vi "AFM Control.vi"() -> ()   [LabVIEW 2020, in "AFM Control.lvclass"]
doc: "Use this VI to help configure your experiment.\n1. Choose Pickering or Not Pickering\n2. Configure the Electrode control to show which electrode is connected to which lockin\n3. Choose a Label for each electrode to configure Krohn Hite amplifier automatically\n4. Easily set all Krohn Hite channels to be \"all ground\" or \"all differential\" mode\n5. Fill out information about you and your device in the lower left corner\n6. When you are finished, or when you want to update the amplifiers, click the \"CREATE OUTPUT\" button located in upper right. Clicking this button will set the amplifiers, Pickering switch (if you have one), and write information to a functional global variable that you can easily read from elsewhere in your program"
uses:
  AFM Control.lvclass
  Typedefs/Instrument--enum.ctl
  AFM Control.lvclass/AFM Control.ctl
  <userlib>/_MGI/File/MGI Create Directory Chain Behavior Enum.ctl
  <vilib>/MakerHub/Toolbox/LMH-Toolbox.lvlib
panel:
  in  "Create Output":bool
  in  "OK":bool
  out "Control Experiment":refnum<class "AFM Control.lvclass">
  in  "Control Experiment":refnum<class "AFM Control.lvclass">
  in  "Tab Control":T1(tab)=enum."LevyLabVIEW output"
  in  "Project & Device Description":string="this is a test"
  in  "Sample":string="TEST"
  in  "Device":string="20191017"
  in  "Instrument":T2=enum."EBL"
  in  "Username":string="Dengyu"
  out "device":string="TEST.20191017"
  out "comments":string="Device: \r  Device Name: TEST.20191017\r  Computer: BLACKPEARL\r  User: Dengyu\r  Instrument: EBL\r  Description: |\r    this is a test\r\rExperiment: \r  Time: 2019-10-18T11:10:03\r  Description: |\rSweep: \r- Loop1: [OFF, 0.000000]\r- Loop2: [OFF, 0.000000]\r- Loop3: [OFF, 0.000000]\r- Loop4: [OFF, 0.000000]\r\rWiring: \r- Electrode 1: Lockin 1, I-, KH1 Channel 1, Differential, 1x, 50k Ohms\r- Electrode 2: Lockin 2, Vsg, KH1 Channel 2, Differential, 1x, 50k Ohms\r- Electrode 4: Lockin 3, V1+, KH1 Channel 3, SE+ (-gnd), 10x, Open\r- Electrode 3: Lockin 4, V1-, KH1 Channel 4, SE+ (-gnd), 10x, Open\r- Electrode 26: Lockin 6, I+, KH1 Channel 6, Differential, 1x, 50k Ohms\r\rLockin: \r  AO: \r  - AO 1: amp = 10.000 mV, DC = 0.000 mV, f = 13.00 Hz, phi = 0.00°, Sine\r  - AO 2: amp = 0.000 mV, DC = 0.000 mV, f = 13.00 Hz, phi = 0.00°, Sine\r  - AO 3: amp = 0.000 mV, DC = 0.000 mV, f = 13.00 Hz, phi = 0.00°, Sine\r  - AO 4: amp = 0.000 mV, DC = 0.000 mV, f = 13.00 Hz, phi = 0.00°, Sine\r  REF: \r  - Lockin 1: f = 13.00 Hz, phi = 0.00°, TC = 0.10 s, order = 2 \r  Sampling: \r  - Fs: 65000.000000\r  - N: 5000\r"
  out "folder":string="G:\\My Drive\\ansom\\Data\\EBL\\TEST.20191017" caption="(\\base path\\project\\device\\ )"
  out "Values have changed":bool
  in  "KH Same Gain":bool
  in  "KH Same Shunt":bool
  out "YAML example":string="description: This is a dummy dataset which mimics smFRET data.\n\nsetup:\n    ## Mandatory fields\n    num_pixels: 2                # using 2 detectors\n    num_spots: 1                 # a single confocal excitation\n    num_spectral_ch: 2           # donor and acceptor detection\n    num_polarization_ch: 1       # no polarization selection\n    num_split_ch: 1              # no beam splitter\n    modulated_excitation: False  # CW excitation, no modulation\n    lifetime: False              # no TCSPC in detection\n\n    ## Optional fields\n    excitation_wavelengths:      # List of excitation wavelenghts\n       - !!float 532e-9\n    excitation_cw:               # List of booleans, True if wavelength is CW\n       - True\n    detection_wavelengths:       # Nominal center wavelength for each for detection ch\n       - !!float 580e-9\n       - !!float 640e-9\n\nsample:\n  sample_name: describe the sample here\n  buffer_name: describe the buffer here\n  dye_names: 'Cy3B, ATTO647N'   # Comma separates names of fluorophores\n\nidentity:\n    author: Author Name\n    author_affiliation: Name of Research Institution\n\nprovenance:\n    filename: 'photon_data.hdf5'\n    software: Acquisition Software Name\n\nphoton_data:\n    timestamps_specs:\n        timestamps_unit: !!float 10e-9  # 10 ns\n    measurement_specs:\n        measurement_type: smFRET\n        detectors_specs:\n            spectral_ch1: [0]  # list of donor's detector IDs\n            spectral_ch2: [1]  # list of acceptor's detector IDs"
  in  "String":string
  # "Lockin"
  # "Krohn Hite"
  # "Other"
  # "Wiring"
  # "Use this VI to help configure your experiment.\n1. Choose Pickering or Not Pickering\n2. Configure the Electrode control to show which electrode is connected to which lockin\n3. Choose a Label for each electrode to configure Krohn Hite amplifier automatically\n4. Easily set all Krohn Hite channels to be \"all ground\" or \"all differential\" mode\n5. Fill out information about you and your device in the lower left corner\n6. When you are finished, or when you want to update the amplifiers, click the \"CREATE OUTPUT\" button located in upper right.\nClicking this button will set the amplifiers, Pickering switch (if you have one), and write information to a functional global variable that you can easily read from elsewhere in your program"
  # "If you want to have new labels for the \"Labels\" field you can type them here"
  # "Not used:"
  # "The magic words are:\nI\nVsg\nVbg\ndV\nV"
  # "Sample"
  # "Krohn Hite"
  # "Lockin"
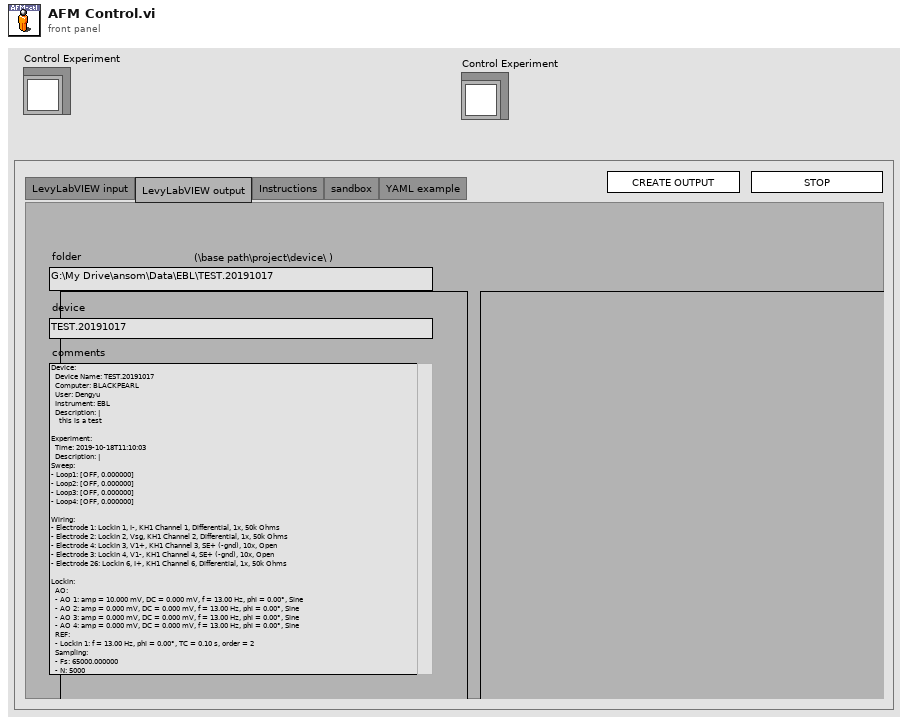
[diagram p1: front panel]
types:
  T1 = enum32{"LevyLabVIEW input", "LevyLabVIEW output", "Instructions", "sandbox", "YAML example"}
  T2 = typedef "AFM Control.lvclass/Instrument--enum.ctl" = enum16{"PPMS", "PPMS2", "MFP3D", "CYPHER", "THz1", "THz2", "MNK", "CF900", "JEOL", "AGILENT", "EBL"}
  T3 = enum32{"invalid app kind", "Development System", "Run Time System", "Student Edition", "Embedded LabVIEW", "Evaluation", "Custom"}
  T4 = enum32{"Invalid", "Standard", "Closed", "Hidden", "Minimized", "Maximized"}
  T5 = typedef "MGI Create Directory Chain Behavior Enum.ctl" = enum16{"Auto Detect", "Path Contains a File", "Path Does Not Contain a File"}
  T6 = typedef "AFM Control.lvclass/Experiment Description--cluster.ctl" = cluster{"User":string, "Device":string, "Device Path":path, "Device Description":string, "Experiment Path":path, "Experiment Description":string, "Instrument":T2}
  T7 = cluster{"Core":cluster{"Current VI Reference":refnum<vi>, "Close Panel on Exit?":bool}, "Control Experiment":refnum<class "AFM Control.lvclass">, "Experiment":T6}
  T8 = cluster{"Current VI Reference":refnum<vi>, "Close Panel on Exit?":bool}
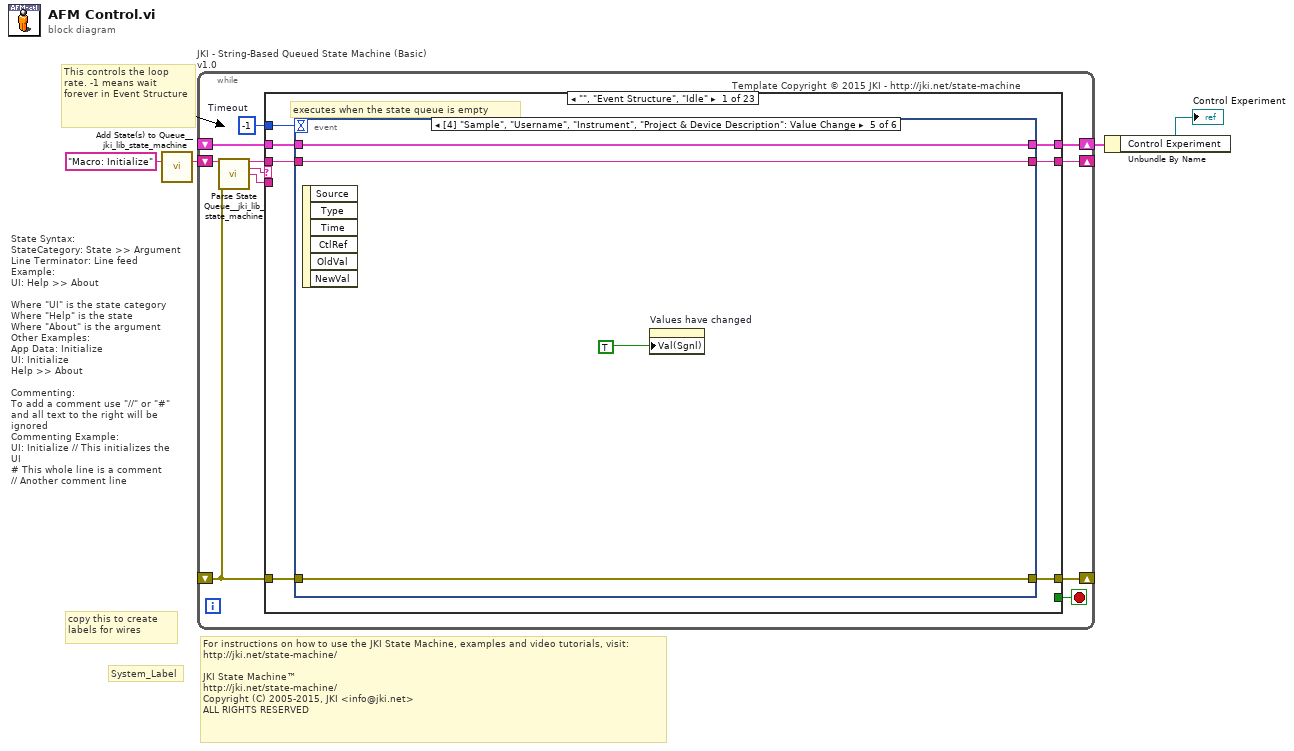
[diagram p0: block diagram]
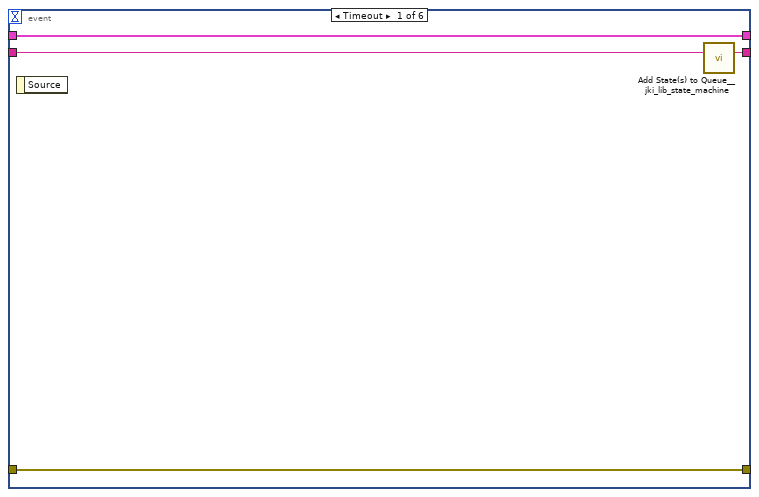
[diagram p2: hidden frame]
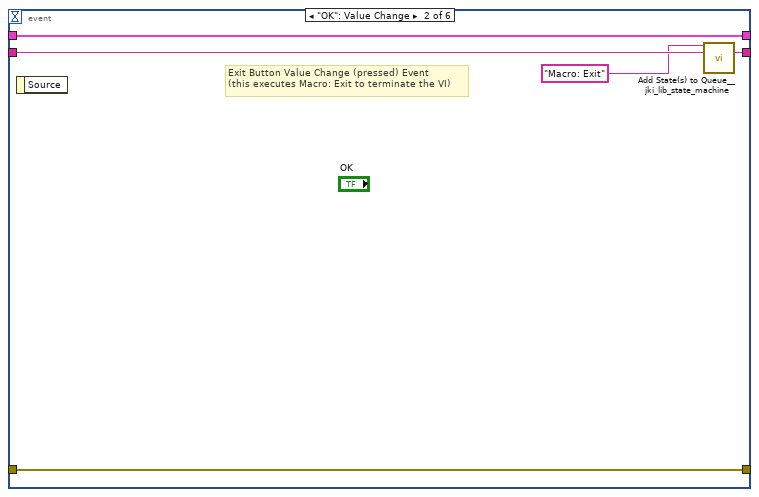
[diagram p3: hidden frame]
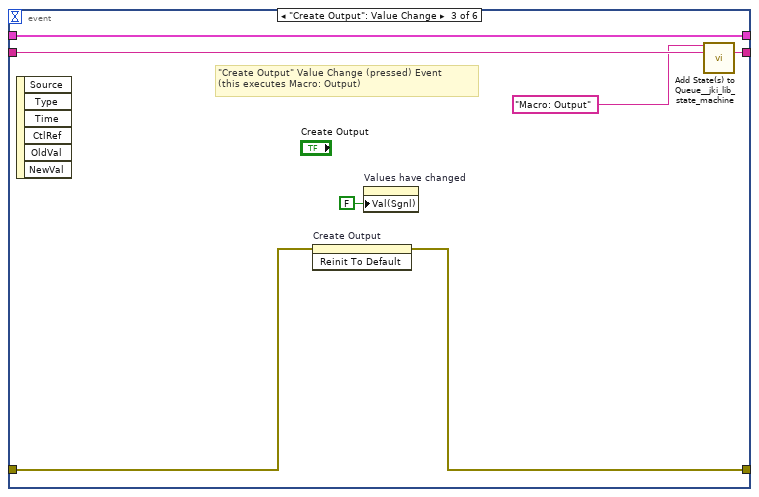
[diagram p4: hidden frame]
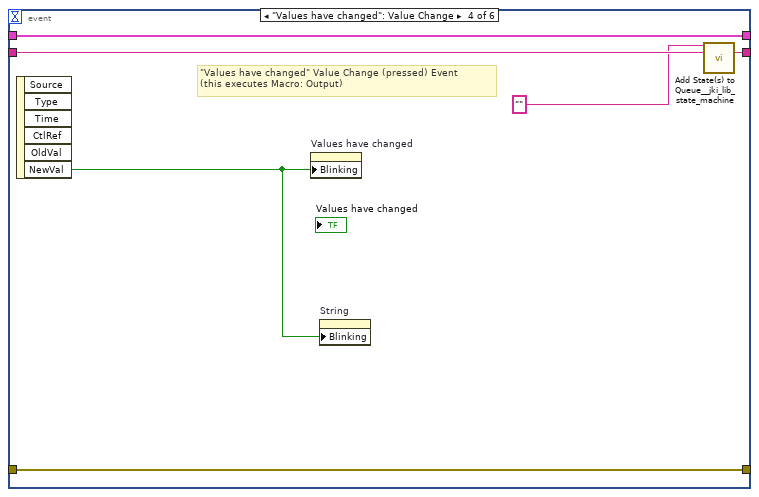
[diagram p5: hidden frame]
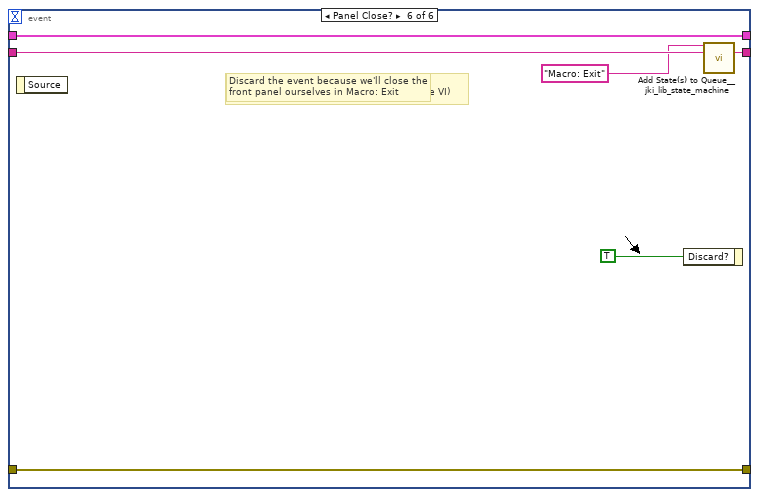
[diagram p6: hidden frame]
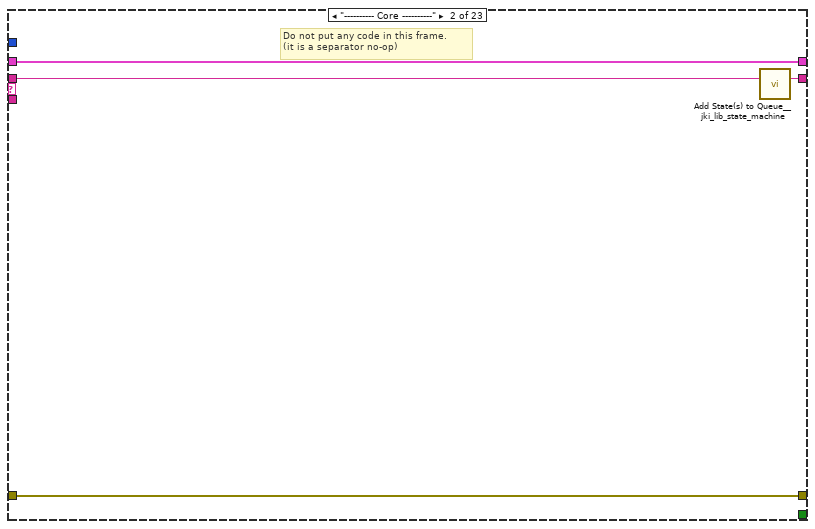
[diagram p7: hidden frame]
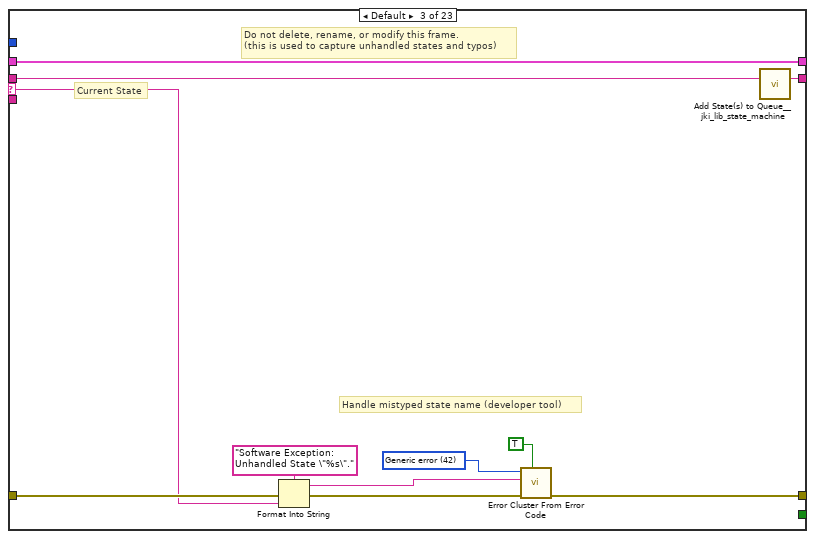
[diagram p8: hidden frame]
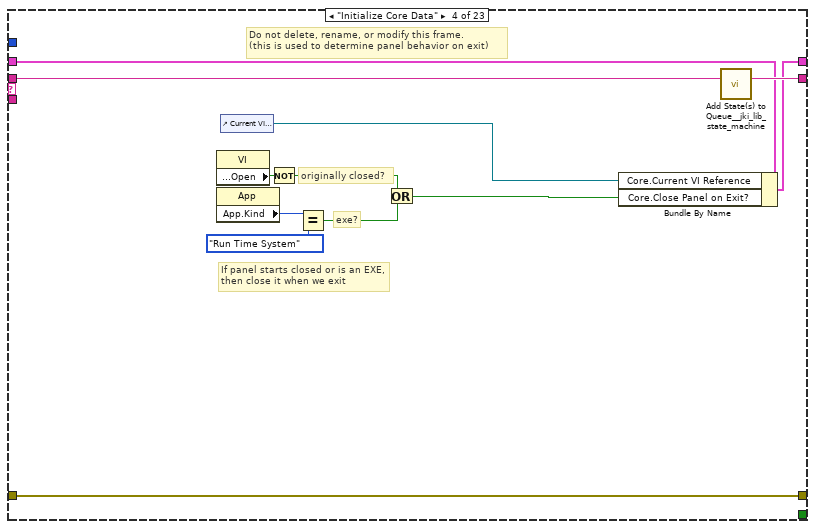
[diagram p9: hidden frame]
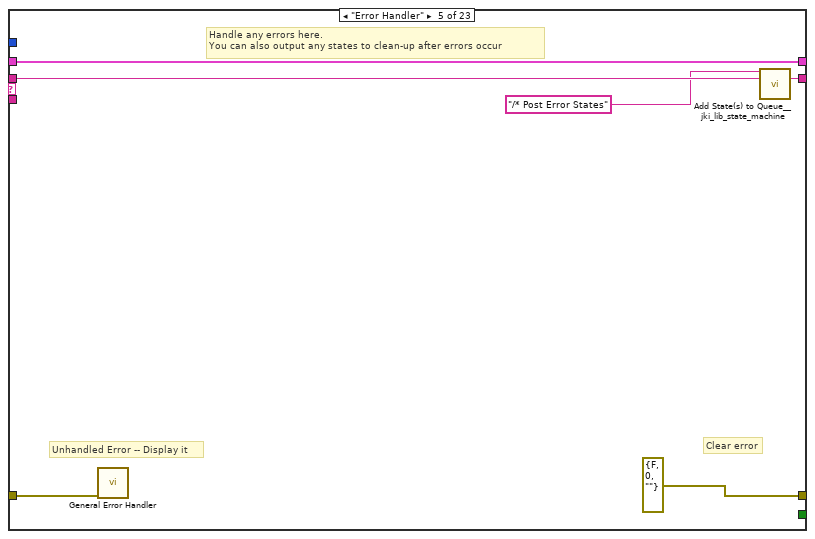
[diagram p10: hidden frame]
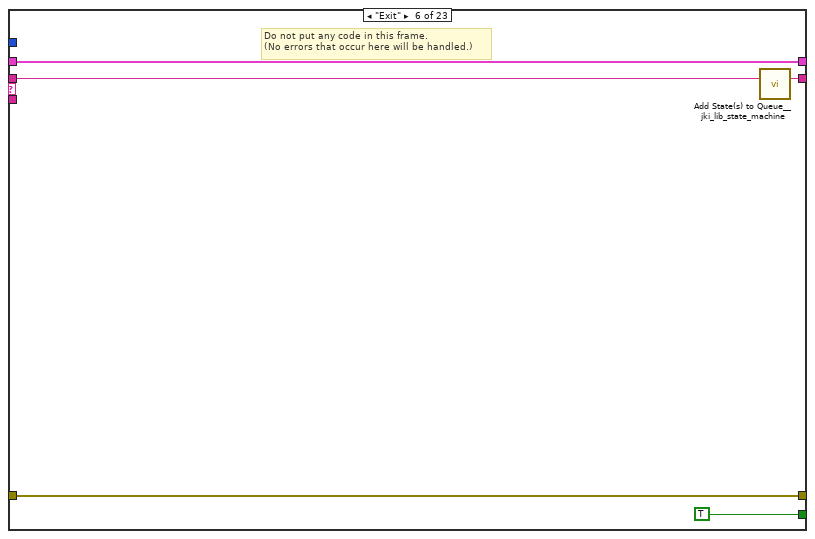
[diagram p11: hidden frame]
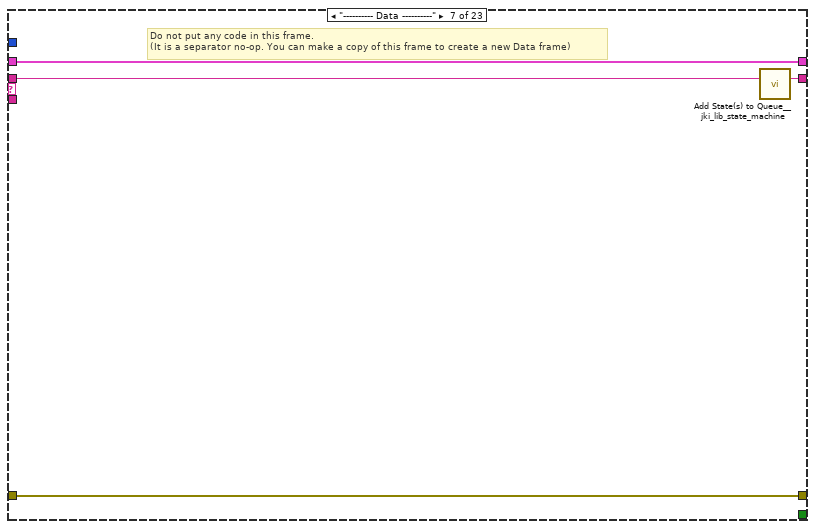
[diagram p12: hidden frame]
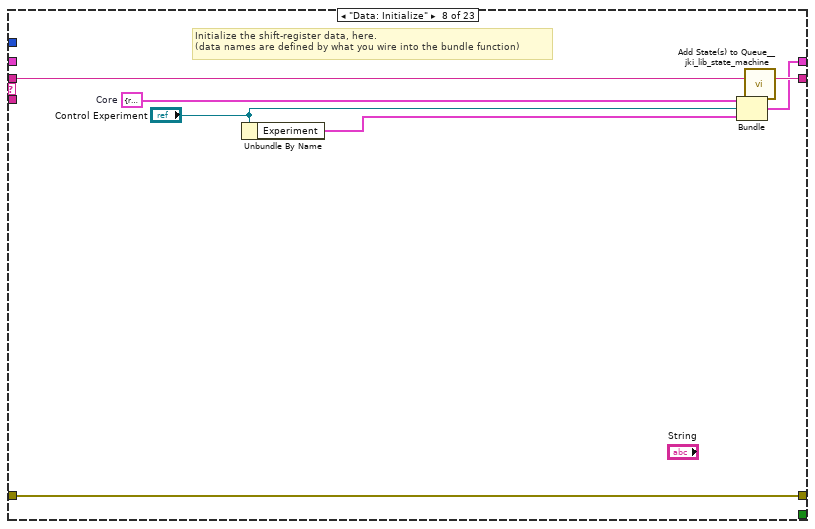
[diagram p13: hidden frame]
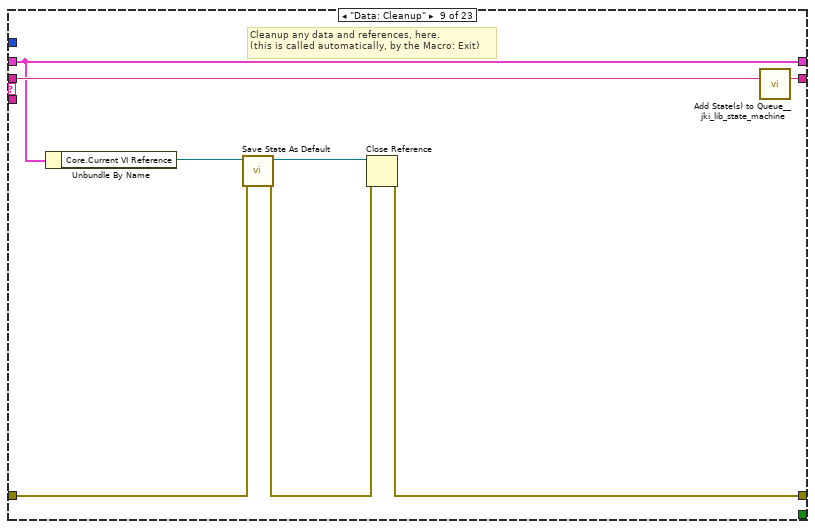
[diagram p14: hidden frame]
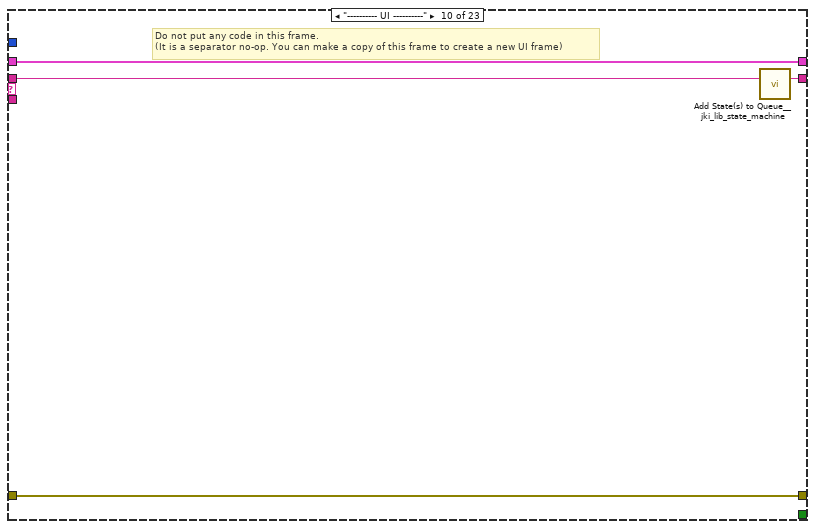
[diagram p15: hidden frame]
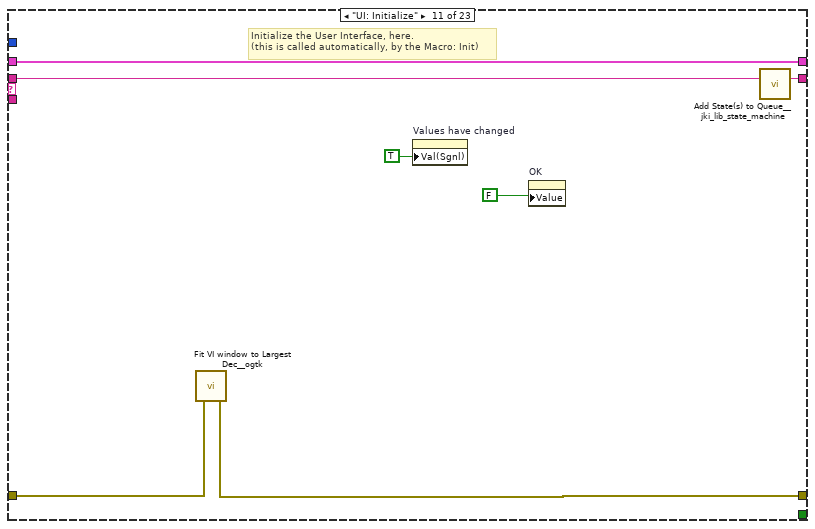
[diagram p16: hidden frame]
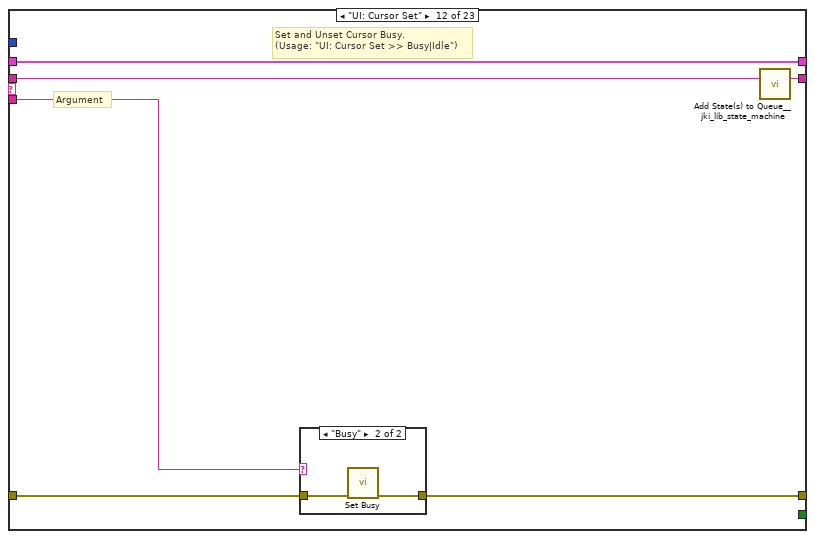
[diagram p17: hidden frame]
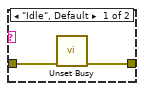
[diagram p18: hidden frame]
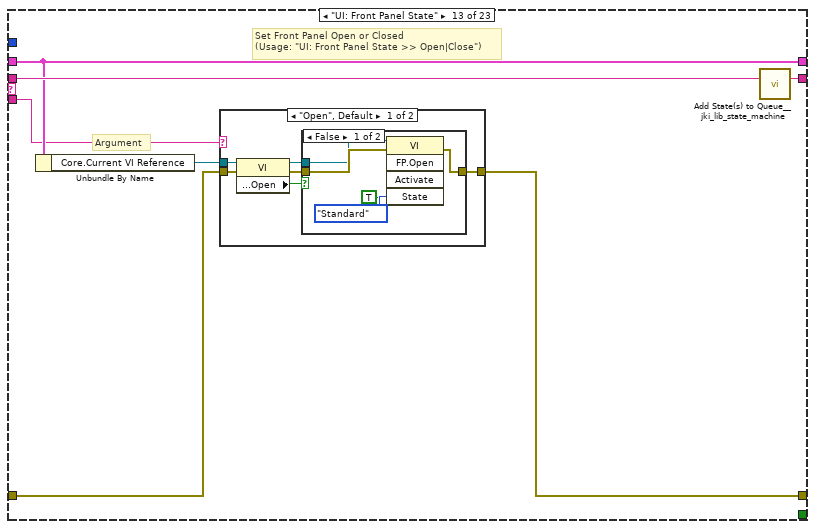
[diagram p19: hidden frame]
diagram:
  # "For instructions on how to use the JKI State Machine, examples and video tutorials, visit:\nhttp://jki.net/state-machine/\n\nJKI State Machine™\nhttp://jki.net/state-machine/\nCopyright (C) 2005-2015, JKI <info@jki.net>\nALL RIGHTS RESERVED"
  # "State Syntax:\nStateCategory: State >> Argument\nLine Terminator: Line feed\nExample:\nUI: Help >> About\n\nWhere \"UI\" is the state category\nWhere \"Help\" is the state\nWhere \"About\" is the argument\nOther Examples:\nApp Data: Initialize\nUI: Initialize\nHelp >> About\n\nCommenting:\nTo add a comment use \"//\" or \"#\" and all text to the right will be ignored\nCommenting Example:\nUI: Initialize // This initializes the UI\n# This whole line is a comment\n// Another comment line"
  # "copy this to create labels for wires"
  # "This controls the loop rate. -1 means wait forever in Event Structure"
  # "System_Label"
  n1 = call <vilib>:"Add State(s) to Queue__jki_lib_state_machine.vi"("State(s) in (\"\")"="Macro: Initialize") -> ("States Out"=w4:string)  [unwired: 14 in]
  n2 = while "JKI - String-Based Queued State Machine (Basic) v1.0" {
    shift-right: [w8] -> w2
    shift-left: _ -> [w7]
    shift-right: [w11] -> _
    shift-left: _ -> [w5]
    shift-right: [w10] -> _
    shift-left: w4 -> [w12]
    stop <- w9 stop-if-true
    w6 = -1  # Timeout
    # "Template Copyright © 2015 JKI - http://jki.net/state-machine"
    n3 = call <vilib>:"Parse State Queue__jki_lib_state_machine.vi"("State Queue"=w12, "Error In (no error)"=w5) -> ("Remaining States"=w14:string, "Current State"=w15:string, "Arguments"=w13:string)  [unwired: 11 in]
    n4 = case shown="\"\", \"Event Structure\", \"Idle\"" w15 {
      selector: w15 -> [_ _ w59 _ _ _ _ _ _ _ _ _ _ _ _ _ _ _ _ _ _ _ _]
      tunnel: w14 -> [w22 w58 w63 w81 w87 w92 w96 w103 w111 w115 w122 w128 w139 w165 w169 w174 w185 w192 w196 w208 w223 w236 w243]
      tunnel: w13 -> [_ _ _ _ _ _ _ _ _ _ _ w123 w133 _ _ _ _ _ _ _ _ _ _]
      tunnel: w7 -> [w20 w55 w61 w72 w84 w90 w93 _ w109 w112 w120 w126 w135 w162 w166 w171 w182 w190 w193 w204 w221 w234 w241]
      tunnel: [w19 w56 w65 w78 errorcluster {"status"=FALSE, "code"=0, "source"=""} ("error out") w89 w94 w100 w108 w113 w116 w124 w136 w163 w167 w172 w183 w187 w194 w206 w211 w227 w239] -> w11
      tunnel: w5 -> [w18 w56 w64 w78 w83 w89 w94 w100 w105 w113 w119 w125 w137 w163 w167 w172 w183 w187 w194 w206 w212 w228 w237]
      tunnel: [w21 w57 w62 w80 w86 w91 w95 w102 w110 w114 w121 w127 w138 w164 w168 w173 w184 w191 w195 w207 w222 w235 w242] -> w10
      tunnel: [_ _ _ _ _ TRUE _ _ _ _ _ _ _ _ _ _ _ _ _ _ _ _ _] -> w9
      tunnel: [w17 w55 w61 w79 w84 w90 w93 w101 w109 w112 w120 w126 w135 w162 w166 w171 w182 w190 w193 w205 w220 w233 w241] -> w8
      tunnel: w6 -> [w16 _ _ _ _ _ _ _ _ _ _ _ _ _ _ _ _ _ _ _ _ _ _]
      frame "", "Event Structure", "Idle" {
        # "executes when the state queue is empty"
        n5 = event shown="[4] \"Sample\", \"Username\", \"Instrument\", \"Project & Device Description\": Value Change" {
          selector: _ -> [_ _ _ _ _ _]
          dyn-events: _ -> [_ _ _ _ _ _]
          timeout: w16 -> [_ _ _ _ _ _]
          tunnel: w22 -> [w26 w31 w38 w44 w46 w54]
          tunnel: [w25 w30 w37 w43 w46 w53] -> w21
          tunnel: w20 -> [w23 w28 w36 w42 w47 w51]
          tunnel: [w24 w29 w33 w40 w48 w52] -> w19
          tunnel: w18 -> [w24 w29 w34 w40 w48 w52]
          tunnel: [w23 w28 w36 w42 w47 w51] -> w17
          event Timeout {
            n6 = event-data() -> ()  [unwired: 1 in, 1 out]
            n7 = call <vilib>:"Add State(s) to Queue__jki_lib_state_machine.vi"("State(s) in (\"\")"=w26) -> ("States Out"=w25:string)  [unwired: 14 in]
          }
          event "OK": Value Change {
            # "Exit Button Value Change (pressed) Event\n(this executes Macro: Exit to terminate the VI)"
            n8 = event-data() -> ()  [unwired: 1 in, 1 out]
            n9 = call <vilib>:"Add State(s) to Queue__jki_lib_state_machine.vi"("State(s) in Front (\"\")"="Macro: Exit", "State(s) in (\"\")"=w31) -> ("States Out"=w30:string)  [unwired: 13 in]
          }
          event "Create Output": Value Change {
            # "\"Create Output\" Value Change (pressed) Event\n(this executes Macro: Output)"
            n10 = event-data() -> ()  [unwired: 1 in, 6 out]
            n11 = invoke on="Create Output" class="Bool" method="Reinit To Default"(error in=w34) -> (error out=w33:errorcluster)  [unwired: 2 in, 2 out]
            n12 = property on="Values have changed" class="Bool (strict)"("Val(Sgnl)"=FALSE ("Value (Signaling)")) -> ()  [unwired: 2 in, 2 out]
            n13 = call <vilib>:"Add State(s) to Queue__jki_lib_state_machine.vi"("State(s) in Front (\"\")"="Macro: Output", "State(s) in (\"\")"=w38) -> ("States Out"=w37:string)  [unwired: 13 in]
          }
          event "Values have changed": Value Change {
            # "\"Values have changed\" Value Change (pressed) Event\n(this executes Macro: Output)"
            n14 = event-data() -> ("NewVal"=w39:bool)  [unwired: 1 in, 5 out]
            n15 = property on="Values have changed" class="Bool (strict)"("Blinking"=w39) -> ()  [unwired: 2 in, 2 out]
            n16 = property on="String" class="Str"("Blinking"=w39) -> ()  [unwired: 2 in, 2 out]
            n17 = call <vilib>:"Add State(s) to Queue__jki_lib_state_machine.vi"("State(s) in Front (\"\")"="", "State(s) in (\"\")"=w44) -> ("States Out"=w43:string)  [unwired: 13 in]
          }
          event "Sample", "Username", "Project & Device Description": Value Change {
            n18 = event-data() -> ()  [unwired: 1 in, 6 out]
            n19 = property on="Values have changed" class="Bool (strict)"("Val(Sgnl)"=TRUE ("Values have changed")) -> ()  [unwired: 2 in, 2 out]
          }
          event Panel Close? {
            # "Discard the event because we'll close the front panel ourselves in Macro: Exit"
            # "Close Panel button (pressed) Event\n(this executes Macro: Exit to terminate the VI)"
            n20 = event-data() -> ()  [unwired: 1 in, 1 out]
            n21 = event-data("Discard?"=TRUE) -> ()  [unwired: 1 in, 1 out]
            n22 = call <vilib>:"Add State(s) to Queue__jki_lib_state_machine.vi"("State(s) in Front (\"\")"="Macro: Exit", "State(s) in (\"\")"=w54) -> ("States Out"=w53:string)  [unwired: 13 in]
          }
        }
      }
      frame "---------- Core ----------" {
        # "Do not put any code in this frame.\n(it is a separator no-op)"
        n23 = call <vilib>:"Add State(s) to Queue__jki_lib_state_machine.vi"("State(s) in (\"\")"=w58) -> ("States Out"=w57:string)  [unwired: 14 in]
      }
      frame Default {
        w68 = 42 items=["No error", "Argument error", "Memory is full", "Out of zone", "End of file", "File already open", "Generic file I/O error", "File not found", "File permission error", "Disk is full", "Duplicate path", "Too many files open", "System feature not enabled", "Resource file not found", "Cannot add resource", "Resource not found", "Image not found", "Image memory error", "Pen does not exist", "Config type invalid", "Config token not found", "Config parse error", "Config memory error", "Bad external code format", "Bad external code offset", "External code not present", "Null window", "Destroy window error", "Null menu", "Print aborted", "Bad print record", "Print driver error", "Windows error during printing", "Memory error during printing", "Print dialog error", "Generic print error", "Invalid device refnum", "Device not found", "Device parameter error", "Device unit error", "Cannot open device", "Device call aborted", "Generic error", "Cancelled by user", "Object ID too low", "Object ID too high", "Object not in heap", "Unknown heap", "Unknown object (invalid DefProc)", "Unknown object (DefProc not in table)", "Message out of range", "Invalid (null) method", "Unknown message", "Manager call not supported", "Bad address", "Network operation in progress", "Network operation timed out", "Connection is busy", "Network attribute not supported", "Network error", "Address in use", "System out of memory", "Connection aborted", "Connection refused", "Not connected", "Already connected", "Connection closed", "Initialization error (interapplication manager)", "Bad occurrence", "Wait on unbound occurrence handler", "Occurrence queue overflow", "Datalog type conflict", "Unused", "Unrecognized type (interapplication manager)", "Memory corrupt", "Failed to make temporary DLL", "Old CIN version", "Drag socket not found", "Failed to load drop-object", "Failed to register OLE object", "Failed to release OLE object", "Format specifier type mismatch", "Unknown format specifier", "Too few format specifiers", "Too many format specifiers", "Scan failed", "Newer CIN version", "Error converting to variant", "Runtime menu error", "Password tampered", "Variant attribute not found", "Incompatible variant data type", "Event data is not available", "Event Store is not present", "Occurrence is not found", "Event Queue is not created", "Event info is not available", "Refnum passed is NULL", "Error retrieving Class GUID", "Error retrieving CoClass GUID", "Error retrieving TypeLib GUID.", "Bad built application magic bytes.", "Specific driver is different from the specific driver associated with the Logical Name.", "There is no session opened to the class driver.", "Max Error", "MAX - Error with config objects", "MAX - Error loading configuration", "MAX - Group not supported"]
        # "Current State"
        # "Do not delete, rename, or modify this frame.\n(this is used to capture unhandled states and typos)"
        # "Handle mistyped state name (developer tool)"
        n24 = Format Into String(format string="Software Exception: Unhandled State \"%s\"." ("message"), error in=w64, w59) -> (resulting string=w67:string, error out=w66:errorcluster)  [unwired: 1 in]
        n25 = call <vilib>:"Error Cluster From Error Code.vi"("show call chain? (False)"=TRUE, "error in (no error)"=w66, "error message (\"\")"=w67, "error code (0)"=w68) -> ("error out"=w65:errorcluster)  [unwired: 5 in]
        n26 = call <vilib>:"Add State(s) to Queue__jki_lib_state_machine.vi"("State(s) in (\"\")"=w63) -> ("States Out"=w62:string)  [unwired: 14 in]
      }
      frame "Initialize Core Data" {
        # "Do not delete, rename, or modify this frame.\n(this is used to determine panel behavior on exit)"
        # "originally closed?"
        # "exe?"
        # "If panel starts closed or is an EXE, then close it when we exit"
        n27 = property class="VI"() -> ("Front Panel.Open"=w77:bool)  [unwired: 2 in, 2 out]
        n28 = property class="App"() -> ("App.Kind"=w76:T3)  [unwired: 2 in, 2 out]
        n29 = control-ref of="Current VI Reference"() -> (w70:refnum<vi>)
        n30 = Not(x=w77) -> (.not. x?=w74:bool)
        n31 = Equal?(x=w76, y=T3."Run Time System" ("Application:Kind")) -> (x = y?=w73:bool)
        n32 = Or(x=w74, y=w73) -> (x .or. y?=w71:bool)
        n33 = Bundle By Name(cluster=w72, "Core.Current VI Reference"=w70, "Core.Close Panel on Exit?"=w71) -> (w79:T7)
        n34 = call <vilib>:"Add State(s) to Queue__jki_lib_state_machine.vi"("State(s) in (\"\")"=w81) -> ("States Out"=w80:string)  [unwired: 14 in]
      }
      frame "Error Handler" {
        # "Unhandled Error -- Display it"
        # "Handle any errors here.\nYou can also output any states to clean-up after errors occur"
        # "Clear error"
        n35 = call <vilib>:"General Error Handler.vi"("error in (no error)"=w83) -> ()  [unwired: 10 in, 5 out]
        n36 = call <vilib>:"Add State(s) to Queue__jki_lib_state_machine.vi"("State(s) in Front (\"\")"="/* Post Error States", "State(s) in (\"\")"=w87) -> ("States Out"=w86:string)  [unwired: 13 in]
      }
      frame "Exit" {
        # "Do not put any code in this frame.\n(No errors that occur here will be handled.)"
        n37 = call <vilib>:"Add State(s) to Queue__jki_lib_state_machine.vi"("State(s) in (\"\")"=w92) -> ("States Out"=w91:string)  [unwired: 14 in]
      }
      frame "---------- Data ----------" {
        # "Do not put any code in this frame.\n(It is a separator no-op. You can make a copy of this frame to create a new Data frame)"
        n38 = call <vilib>:"Add State(s) to Queue__jki_lib_state_machine.vi"("State(s) in (\"\")"=w96) -> ("States Out"=w95:string)  [unwired: 14 in]
      }
      frame "Data: Initialize" {
        w99 = T8 {"Current VI Reference"=refnum, "Close Panel on Exit?"=FALSE}  # Core
        # "Initialize the shift-register data, here.\n(data names are defined by what you wire into the bundle function)"
        n39 = Unbundle By Name("Control Experiment") -> ("Experiment"=w97:T6)
        n40 = Bundle("Core"=w99, "Control Experiment"="Control Experiment", "Experiment"=w97) -> (w101:T7)  [unwired: 1 in]
        n41 = call <vilib>:"Add State(s) to Queue__jki_lib_state_machine.vi"("State(s) in (\"\")"=w103) -> ("States Out"=w102:string)  [unwired: 14 in]
      }
      frame "Data: Cleanup" {
        # "Cleanup any data and references, here.\n(this is called automatically, by the Macro: Exit)"
        n42 = Unbundle By Name(w109) -> ("Core.Current VI Reference"=w107:refnum<vi>)
        n43 = call <vilib>:"Save State As Default.vi"("Error In"=w105, "Target VI"=w107) -> ("Error Out"=w104:errorcluster, "Target VI"=w106:refnum<vi>)  [unwired: 8 in]
        n44 = Close Reference(reference=w106, error in (no error)=w104) -> (error out=w108:errorcluster)
        n45 = call <vilib>:"Add State(s) to Queue__jki_lib_state_machine.vi"("State(s) in (\"\")"=w111) -> ("States Out"=w110:string)  [unwired: 14 in]
      }
      frame "---------- UI ----------" {
        # "Do not put any code in this frame.\n(It is a separator no-op. You can make a copy of this frame to create a new UI frame)"
        n46 = call <vilib>:"Add State(s) to Queue__jki_lib_state_machine.vi"("State(s) in (\"\")"=w115) -> ("States Out"=w114:string)  [unwired: 14 in]
      }
      frame "UI: Initialize" {
        # "Initialize the User Interface, here.\n(this is called automatically, by the Macro: Init)"
        n47 = call <userlib>:"Fit VI window to Largest Dec__ogtk.vi"("error in (no error)"=w119) -> ("error out"=w116:errorcluster)  [unwired: 5 in, 1 out]
        n48 = property on="Values have changed" class="Bool (strict)"("Val(Sgnl)"=TRUE ("Blinking")) -> ()  [unwired: 2 in, 2 out]
        n49 = property on="OK" class="Bool (strict)"("Value"=FALSE ("Blinking")) -> ()  [unwired: 2 in, 2 out]
        n50 = call <vilib>:"Add State(s) to Queue__jki_lib_state_machine.vi"("State(s) in (\"\")"=w122) -> ("States Out"=w121:string)  [unwired: 14 in]
      }
      frame "UI: Cursor Set" {
        # "Argument"
        # "Set and Unset Cursor Busy.\n(Usage: \"UI: Cursor Set >> Busy|Idle\")"
        n51 = case shown="\"Busy\"" w123 {
          tunnel: w125 -> [w130 w132]
          tunnel: [w129 w131] -> w124
          frame "Idle", Default {
            n52 = call <vilib>:"Unset Busy.vi"("error in (no error)"=w130) -> ("error out"=w129:errorcluster)  [unwired: 10 in]
          }
          frame "Busy" {
            n53 = call <vilib>:"Set Busy.vi"("error in (no error)"=w132) -> ("error out"=w131:errorcluster)  [unwired: 9 in, 1 out]
          }
        }
        n54 = call <vilib>:"Add State(s) to Queue__jki_lib_state_machine.vi"("State(s) in (\"\")"=w128) -> ("States Out"=w127:string)  [unwired: 14 in]
      }
      frame "UI: Front Panel State" {
        # "Argument"
        # "Set Front Panel Open or Closed\n(Usage: \"UI: Front Panel State >> Open|Close\")"
        n55 = Unbundle By Name(w135) -> ("Core.Current VI Reference"=w134:refnum<vi>)
        n56 = case shown="\"Open\", Default" w133 {
          tunnel: w137 -> [w143 w156]
          tunnel: [w145 w157] -> w136
          tunnel: w134 -> [w144 w154]
          frame "Open", Default {
            n57 = property class="VI"(reference=w144, error in=w143) -> (reference out=w141:refnum<vi>, error out=w142:errorcluster, "Front Panel.Open"=w140:bool)
            n58 = case shown="False" w140 {
              tunnel: [w148 w151] -> w145
              tunnel: w142 -> [w147 w151]
              tunnel: w141 -> [w146 _]
              frame False {
                n59 = invoke class="VI" method="FP.Open"(reference=w146, error in=w147, "Activate"=TRUE, "State"=T4."Standard") -> (error out=w148:errorcluster)  [unwired: 1 in, 4 out]
              }
              frame True {
              }
            }
          }
          frame "Close" {
            n60 = property class="VI"(reference=w154, error in=w156) -> (reference out=w153:refnum<vi>, error out=w155:errorcluster, "Front Panel.Open"=w152:bool)
            n61 = case shown="True" w152 {
              tunnel: [w158 w161] -> w157
              tunnel: w155 -> [w158 w160]
              tunnel: w153 -> [_ w159]
              frame False {
              }
              frame True {
                n62 = invoke class="VI" method="FP.Close"(reference=w159, error in=w160) -> (error out=w161:errorcluster)  [unwired: 1 in, 2 out]
              }
            }
          }
        }
        n63 = call <vilib>:"Add State(s) to Queue__jki_lib_state_machine.vi"("State(s) in (\"\")"=w139) -> ("States Out"=w138:string)  [unwired: 14 in]
      }
      frame "UI: Buttons" {
        # "Do not put any code in this frame.\n(It is a separator no-op. You can make a copy of this frame to create a new UI frame)"
        n64 = call <vilib>:"Add State(s) to Queue__jki_lib_state_machine.vi"("State(s) in (\"\")"=w165) -> ("States Out"=w164:string)  [unwired: 14 in]
      }
      frame "---------- Macro ----------" {
        # "Do not put any code in this frame.\n(It is a separator no-op. You can make a copy of this frame to create a new Macro frame)"
        n65 = call <vilib>:"Add State(s) to Queue__jki_lib_state_machine.vi"("State(s) in (\"\")"=w169) -> ("States Out"=w168:string)  [unwired: 14 in]
      }
      frame "Macro: Initialize" {
        w170 = "Data: Initialize\nInitialize Core Data\nUI: Initialize\nUI: Front Panel State >> Open"  # Data: Initialize Initialize Core Data UI: Initialize UI: Front Panel State >> Open
        # "Initialization Macro\n(This is called once, when the VI starts)"
        n66 = call <vilib>:"Add State(s) to Queue__jki_lib_state_machine.vi"("State(s) in Front (\"\")"=w170, "State(s) in (\"\")"=w174) -> ("States Out"=w173:string)  [unwired: 13 in]
      }
      frame "Macro: Exit" {
        # "Exit Macro\n(This is called once, when the VI exits)"
        n67 = Unbundle By Name(w182) -> ("Core.Close Panel on Exit?"=w181:bool)
        n68 = property on="OK" class="Bool (strict)"("Value"=FALSE ("Blinking")) -> ()  [unwired: 2 in, 2 out]
        n69 = Select(t="UI: Front Panel State >> Close", s=w181, f="") -> (s? t:f=w178:string)
        n70 = call <vilib>:"Add State(s) to Queue__jki_lib_state_machine.vi"("State(s) in (\"\")"=w178, "State(s) at Back (\"\")"="Data: Cleanup\nExit") -> ("States Out"=w176:string)  [unwired: 13 in]
        n71 = call <vilib>:"Add State(s) to Queue__jki_lib_state_machine.vi"("State(s) in Front (\"\")"=w176, "State(s) in (\"\")"=w185) -> ("States Out"=w184:string)  [unwired: 13 in]
      }
      frame "Macro: Output" {
        n72 = call <vilib>:"Add State(s) to Queue__jki_lib_state_machine.vi"("State(s) in Front (\"\")"="Metadata: Update Experiment Description\nMetadata: build path" ("State(s) in Front (\"\")"), "State(s) at Back (\"\")"="Metadata: Update Comments\nMetadata: Update FGV" ("State(s) in Front (\"\")")) -> ("States Out"=w188:string)  [unwired: 13 in]
        n73 = call <vilib>:"Add State(s) to Queue__jki_lib_state_machine.vi"("State(s) in Front (\"\")"=w188, "State(s) in (\"\")"=w192) -> ("States Out"=w191:string)  [unwired: 13 in]
      }
      frame "---------- Metadata ----------" {
        n74 = call <vilib>:"Add State(s) to Queue__jki_lib_state_machine.vi"("State(s) in (\"\")"=w196) -> ("States Out"=w195:string)  [unwired: 14 in]
      }
      frame "Metadata: Update Experiment Description" {
        n75 = Concatenate Strings("Sample", "." ("string"), "Device") -> (w200:string)
        n76 = Bundle By Name(cluster=w204, "Experiment.Device"=w200, "Experiment.User"="Username", "Experiment.Device Description"="Project & Device Description", "Experiment.Instrument"="Instrument") -> (w205:T7)
        n77 = call <vilib>:"Add State(s) to Queue__jki_lib_state_machine.vi"("State(s) in (\"\")"=w208) -> ("States Out"=w207:string)  [unwired: 14 in]
      }
      frame "Metadata: build path" {
        w218 = path "G:/My Drive/ansom/Data"  # Default Path
        n78 = Unbundle By Name(w221) -> ("Experiment.Instrument"=w217:T2, "Experiment.Device"=w215:string)
        "device" <- w215
        n79 = Format Into String(w217) -> (resulting string=w216:string)  [unwired: 3 in, 1 out]
        n80 = Build Path(base path=w218, name or relative path=w216) -> (appended path=w219:path)
        n81 = Build Path(base path=w219, name or relative path=w215) -> (appended path=w214:path)
        n82 = call <userlib>:"MGI Create Directory Chain.vi"("Error In"=w212, "File Presence (Auto Detect)"=MGI_Create_Directory_Chain_Behavior_Enum."Path Does Not Contain a File", "Path"=w214) -> ("Error Out"=w211:errorcluster, "Duplicate Path"=w213:path)  [unwired: 7 in]
        n83 = Path To String(path=w213) -> (string=→"folder":string)
        n84 = Bundle By Name(cluster=w221, "Experiment.Device Path"=w213) -> (w220:T7)
        n85 = call <vilib>:"Add State(s) to Queue__jki_lib_state_machine.vi"("State(s) in (\"\")"=w223) -> ("States Out"=w222:string)  [unwired: 14 in]
      }
      frame "Metadata: Update Comments" {
        # "error 63 occurs when\nthe lockin isn't running\nI think we can clear here?"
        n86 = Unbundle By Name(w234) -> ("Control Experiment"=w230:refnum<class "AFM Control.lvclass">)
        n87 = call "Generate Comments.vi"("error in (no error)"=w228, "AFM Control"=w230) -> ("error out"=w224:errorcluster, "AFM Control out"=w229:refnum<class "AFM Control.lvclass">)  [unwired: 6 in, 1 out]
        n88 = call <vilib>:"Clear Errors.vi"("error in (no error)"=w224, "specific error code to clear (0: all)"=63) -> ("error out"=w225:errorcluster)  [unwired: 4 in, 1 out]
        n89 = call "Read Comments.vi"("error in (no error)"=w225, "AFM Control"=w229) -> ("error out"=w227:errorcluster, "Comments"=→"comments":string, "AFM Control out"=w231:refnum<class "AFM Control.lvclass">)  [unwired: 7 in]
        n90 = Bundle By Name(cluster=w234, "Control Experiment"=w231) -> (w233:T7)
        n91 = call <vilib>:"Add State(s) to Queue__jki_lib_state_machine.vi"("State(s) in (\"\")"=w236) -> ("States Out"=w235:string)  [unwired: 14 in]
      }
      frame "Metadata: Update FGV" {
        n92 = Unbundle By Name(w241) -> ("Control Experiment"=w238:refnum<class "AFM Control.lvclass">)
        n93 = call "AFM Control FGV.vi"("Function"=enum16{"read", "write"}."write", "error in (no error)"=w237, "AFM Control"=w238) -> ("error out"=w239:errorcluster)  [unwired: 7 in, 1 out]
        n94 = call <vilib>:"Add State(s) to Queue__jki_lib_state_machine.vi"("State(s) in (\"\")"=w243) -> ("States Out"=w242:string)  [unwired: 14 in]
      }
    }
  }
  n95 = Unbundle By Name(w2) -> ("Control Experiment"=→"Control Experiment":refnum<class "AFM Control.lvclass">)
